vi "Switching Levels Logic Test.vi"() -> ()   [LabVIEW 2018, in "Elevator.lvlib" / "Elevator.lvclass"]
uses:
  Elevator.lvclass
  Controls/Elevator Position.ctl
  Elevator.lvclass/Elevator.ctl
panel:
  in  "Switch to Hatch":bool
  out "Cargo/Hatch":T1=enum."C0, Cargo Ground"
  in  "Up":bool
  in  "Down":bool
  in  "Switch to cargo":bool
  in  "stop":bool
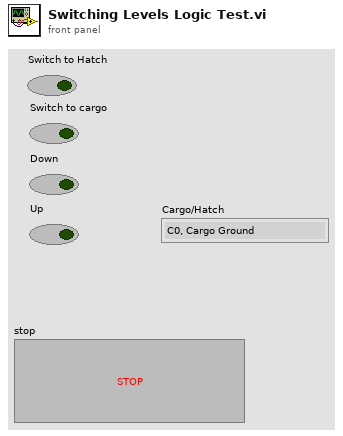
[diagram p1: front panel]
types:
  T1 = typedef "Elevator.lvlib/Elevator.lvclass/Elevator Position.ctl" = enum16{"CS, Cargo Ship Cargo", "C0, Cargo Ground", "C1, LV1 Cargo", "C2, LV2 Cargo", "C3, LV3 Cargo", "H0, LV1 Hatch", "H1, LV2 Hatch", "H2, LV3 Hatch"}
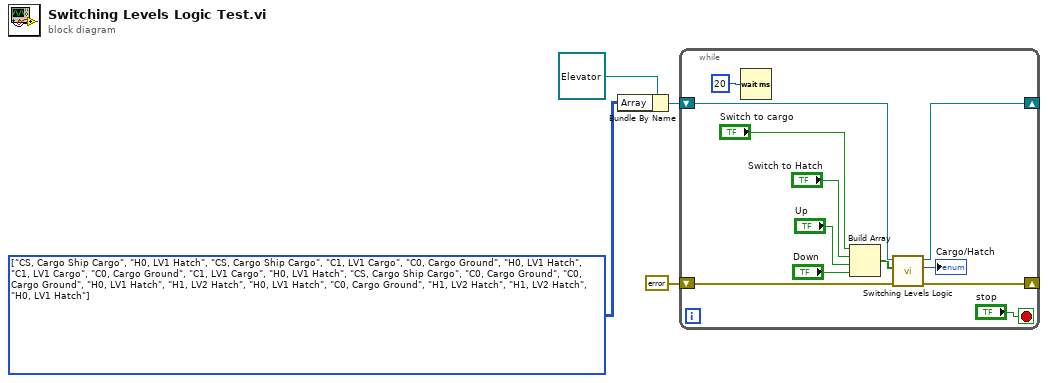
[diagram p0: block diagram]
diagram:
  w1 = T1[][] [[enum."CS, Cargo Ship Cargo", enum."H0, LV1 Hatch", enum."CS, Cargo Ship Cargo", enum."C1, LV1 Cargo"], [enum."C0, Cargo Ground", enum."H0, LV1 Hatch", enum."C1, LV1 Cargo", enum."C0, Cargo Ground"], [enum."C1, LV1 Cargo", enum."H0, LV1 Hatch", enum."CS, Cargo Ship Cargo", enum."C0, Cargo Ground"], [enum."C0, Cargo Ground", enum."H0, LV1 Hatch", enum."H1, LV2 Hatch", enum."H0, LV1 Hatch"], [enum."C0, Cargo Ground", enum."H1, LV2 Hatch", enum."H1, LV2 Hatch", enum."H0, LV1 Hatch"]] items=["CS, Cargo Ship Cargo", "C0, Cargo Ground", "C1, LV1 Cargo", "C2, LV2 Cargo", "C3, LV3 Cargo", "H0, LV1 Hatch", "H1, LV2 Hatch", "H2, LV3 Hatch"] ("Array")
  n1 = Bundle By Name(cluster=refnum<class "Elevator.lvclass"> refnum ("Elevator.lvlib:Elevator.lvclass"), "Array"=w1) -> (w2:refnum<class "Elevator.lvclass">)
  n2 = while {
    shift-right: [w15] -> _
    shift-left: w2 -> [w16]
    shift-right: [w12] -> _
    shift-left: errorcluster {"status"=FALSE, "code"=0, "source"=""} ("error in (no error)") -> [w13]
    stop <- "stop" stop-if-true
    n3 = Wait (ms)(milliseconds to wait=u32 20) -> ()  [unwired: 1 out]
    n4 = Build Array("Switch to cargo", "Switch to Hatch", "Up", "Down") -> (w5:bool[])
    n5 = call "Switching Levels Logic.vi"("error in (no error)"=w13, "buttons"=w5, "Elevator in"=w16) -> ("error out"=w12:errorcluster, "Cargo/Hatch"=→"Cargo/Hatch":T1, "Elevator out"=w15:refnum<class "Elevator.lvclass">)  [unwired: 6 in]
  }
